vi "Get All RFmx VNA Sessions.vi"(0 "TSM Context":T1, 11 "error in":errorcluster) -> (4 "RFmx VNA Sessions":refnum<k21>[](array[refnum]), 15 "error out":errorcluster)   [LabVIEW 2023, in "RFCalAndFixtureCharact.Common.lvlib"]
uses:
  <vilib>/NI_TestStand_SemiconductorModule/NI_TestStand_Semiconductor_Module.lvlibp/PinMap/General/SemiconductorModuleContext.ctl
  Global Data Id Prefix.vi
  RFCalAndFixtureCharact.Common.lvlib
  <vilib>/NI_TestStand_SemiconductorModule/NI_TestStand_Semiconductor_Module.lvlibp
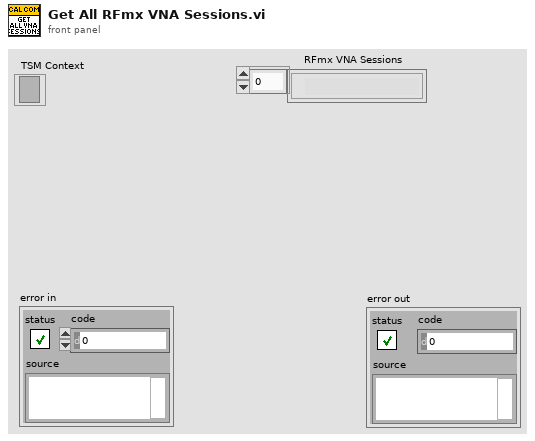
[diagram p1: front panel]
types:
  T1 = typedef "NI_TestStand_Semiconductor_Module.lvlibp/SemiconductorModuleContext.ctl" = refnum<k7>
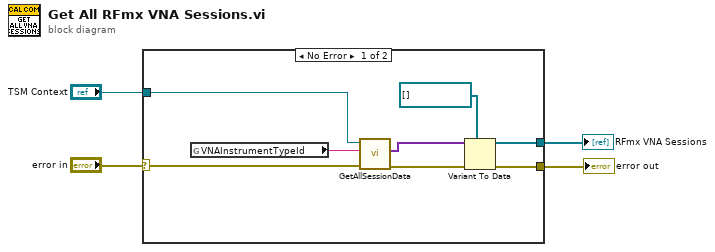
[diagram p0: block diagram]
diagram:
  n1 = case shown="No Error" "error in" {
    selector: "error in" -> [w10 w13]
    tunnel: "TSM Context" -> [w12 _]
    tunnel: [w7 w13] -> w3
    tunnel: [w6 _] -> w1
    frame No Error {
      n2 = global read "Global Data Id Prefix.vi" "VNAInstrumentTypeId"() -> (w11:string)
      n3 = call <vilib>:"GetAllSessionData.vi"("error in (no error)"=w10, "Instrument Type Id"=w11, "Semiconductor Module Context"=w12) -> ("error out"=w8:errorcluster, "Session Data"=w9:variant[])  [unwired: 4 in, 3 out]
      n4 = Variant To Data(error in=w8, type=refnum<k21>[] [] ("RFmx VNA Sessions"), Variant=w9) -> (data=w6:refnum<k21>[], error out=w7:errorcluster)
    }
    frame Error {
    }
  }
  "error out" <- w3
  "RFmx VNA Sessions" <- w1
